vi "PV_Boost.vi"(0 "i_pv(k-1)":fxp<+,24,4>, 1 "D":fxp<+,20,0>, 3 "r_V(G)":fxp<+,25,5>=20.961105346679688, 5 "v_pv(k-1)":fxp<+,26,6>, 7 "vB(k-1)_op":fxp<+,28,8>, 9 "i_L_P(k-1)":fxp<+/-,27,7>, 11 "e":bool, 12 "vB(k-1)":fxp<+,28,8>, 14 "r_I(G)":fxp<+,20,0>=3.147125244140625e-05) -> (4 "i_pv(k)":fxp<+,24,4>, 6 "v_pv(k)":fxp<+,26,6>, 8 "vB(k)_op":fxp<+,28,8>, 10 "i_L_P(k)":fxp<+/-,27,7>, 15 "Io":fxp<+/-,25,5>)   [LabVIEW 2015]
uses:
  <vilib>/rvi/FXPMathLib/FxpSub/XNode/nifxpmath_Sub.xnode
  <vilib>/rvi/FXPMathLib/FxpMul/XNode/nifxpmath_Multiplier.xnode
  <vilib>/rvi/FXPMathLib/FxpAdd/XNode/nifxpmath_Add.xnode
  <vilib>/rvi/FXPMathLib/sim/FxpSim.dll
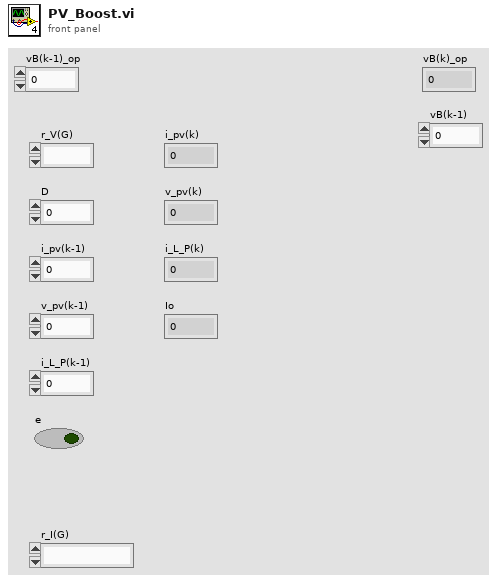
[diagram p1: front panel]
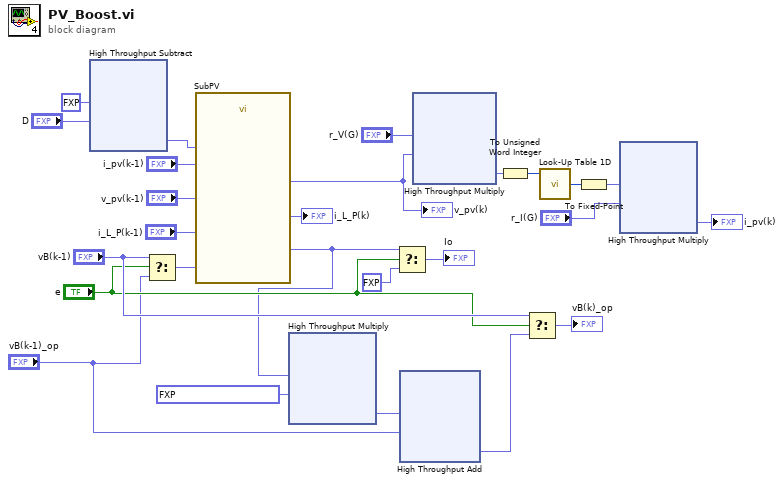
[diagram p0: block diagram]
diagram:
  n1 = xnode "High Throughput Subtract"("x"=fxp<+,1,1> 1.0, "y"="D") -> ("x-y"=w10:fxp<+,20,0>)
  n2 = Select(t="vB(k-1)", s="e", f="vB(k-1)_op") -> (s? t:f=w25:fxp<+,28,8>)
  n3 = call "SubPV.vi"("v_DC(k-1)"=w25, "1-D_P"=w10, "v_pv(k-1)"="v_pv(k-1)", "i_pv(k-1)"="i_pv(k-1)", "i_L_P(k-1)"="i_L_P(k-1)") -> ("i_P"=w3:fxp<+/-,25,5>, "i_L_P(k)"=→"i_L_P(k)":fxp<+/-,27,7>, "v_pv(k)"=w19:fxp<+,26,6>)  [unwired: 12 in]
  "v_pv(k)" <- w19
  n4 = xnode ("High Throughput Multiply")("x"=w3, "y"=fxp<+,20,0> 0.5957450866699219) -> ("x*y"=w4:fxp<+/-,45,5>)
  n5 = Select(t=w3, s="e", f=fxp<+/-,25,5> 0.0) -> (s? t:f=→"Io":fxp<+/-,25,5>)
  n6 = xnode ("High Throughput Add")("x"=w4, "y"="vB(k-1)_op") -> ("x+y"=w5:fxp<+,28,8>)
  n7 = xnode ("High Throughput Multiply")("x"="r_V(G)", "y"=w19) -> ("x*y"=w16:fxp<+,10,10>)
  n8 = To Unsigned Word Integer(number=w16) -> (unsigned 16bit integer=w17:u16)
  n9 = Select(t="vB(k-1)", s="e", f=w5) -> (s? t:f=→"vB(k)_op":fxp<+,28,8>)
  n10 = call "Look-Up Table 1D"("address"=w17) -> ("data out"=w15:u16)  [unwired: 8 in]
  n11 = To Fixed-Point(number=w15) -> (fixed-point=w14:fxp<+,16,16>)  [unwired: 1 in]
  n12 = xnode ("High Throughput Multiply")("x"=w14, "y"="r_I(G)") -> ("x*y"=→"i_pv(k)":fxp<+,24,4>)
